vi "Destroy UI Events.vi"(11 "ABD Panel in":refnum<class "ABD Panel.lvclass">) -> ()   [LabVIEW 2021, in "ABD Panel.lvclass"]
uses:
  ABD Panel.lvclass
  ABD Panel.lvclass/ABD Panel.ctl
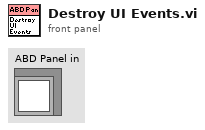
[diagram p1: front panel]
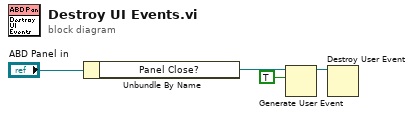
[diagram p0: block diagram]
diagram:
  n1 = Unbundle By Name("ABD Panel in") -> ("Panel Close?"=w1:refnum<user-event>)
  n2 = Generate User Event(user event=w1, event data cluster=TRUE ("event data")) -> (user event out=w3:refnum<user-event>)  [unwired: 2 in, 1 out]
  n3 = Destroy User Event(user event=w3) -> ()  [unwired: 1 in, 1 out]
